vi "SENS_IF_GAIN_ALL_STAT.vi"(0 "VISA IN":refnum<visa-resource-name>, 1 "AUTO or MANUAL":string(combo)="AUTO", 5 "error in":errorcluster, 7 "Channel":i32) -> (14 "VISA Out":refnum<visa-resource-name>, 19 "error out":errorcluster)   [LabVIEW 2018, in "PNA-X.lvlib"]
doc: "SENSe<cnum>:IF:GAIN:ALL[:STATe] <char> \n(Write only) Sets the gain state for ALL receivers to Auto or Manual. \nParameters \n<cnum> Existing channel number to manipulate. If unspecified, <cnum> is set to 1. \n<char> Choose from AUTO or MANUAL \nExamples SENS:IF:GAIN:ALL AUTO \nsense:if:gain:all:state manual \nQuery Syntax Not Applicable \nReturn Type Character \nDefault AUTO"
uses:
  PNA-X.lvlib
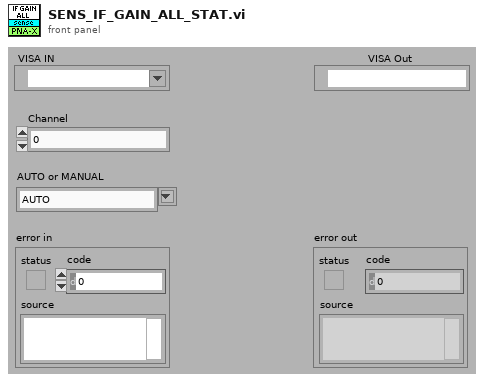
[diagram p1: front panel]
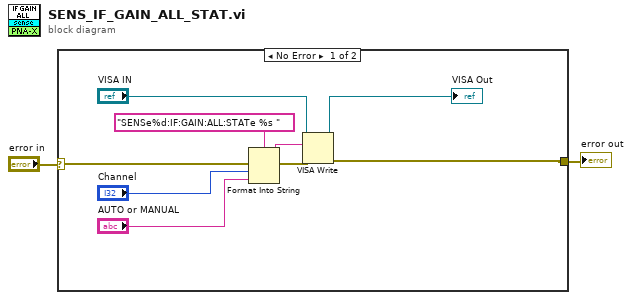
[diagram p0: block diagram]
diagram:
  n1 = case shown="No Error" "error in" {
    selector: "error in" -> [w11 w12]
    tunnel: [w6 w12] -> w1
    frame No Error {
      n2 = Format Into String(format string="SENSe%d:IF:GAIN:ALL:STATe %s " ("Cmdline"), error in=w11, "Channel", "AUTO or MANUAL") -> (resulting string=w9:string, error out=w10:errorcluster)  [unwired: 1 in]
      n3 = VISA Write(VISA resource name="VISA IN", write buffer=w9, error in (no error)=w10) -> (VISA resource name out=→"VISA Out":refnum<visa-resource-name>, error out=w6:errorcluster)  [unwired: 1 out]
    }
    frame Error {
    }
  }
  "error out" <- w1
